vi "robo_getVersion.vi"(0 "VISA资源名称":refnum<visa-resource-name>, 1 "错误输入（无错误）":errorcluster) -> (2 "VISA资源名称输出":refnum<visa-resource-name>, 3 "读取缓冲区":string, 4 "错误输出":errorcluster)   [LabVIEW 2017]
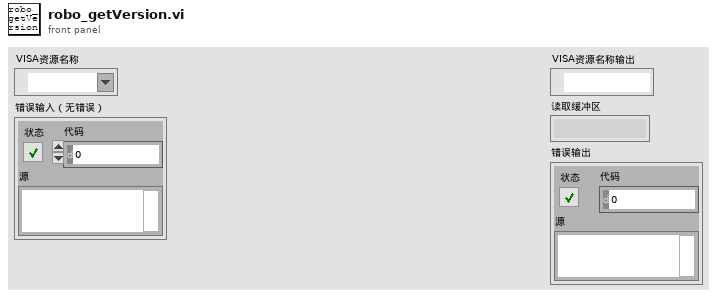
[diagram p1: front panel]
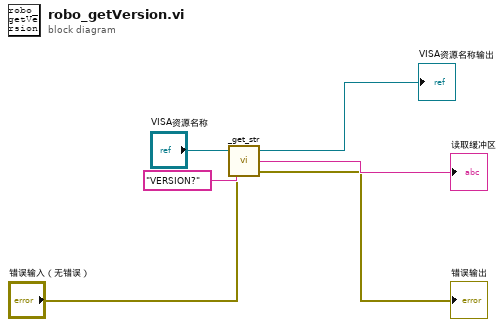
[diagram p0: block diagram]
diagram:
  n1 = call "_get_str.vi"("错误输入（无错误）"="错误输入（无错误）", "写入缓冲区"="VERSION?", "VISA资源名称"="VISA资源名称") -> ("错误输出"=→"错误输出":errorcluster, "读取缓冲区"=→"读取缓冲区":string, "VISA资源名称输出"=→"VISA资源名称输出":refnum<visa-resource-name>)
